vi "To String (Numeric).vi"(7 "enable LabVIEW extensions? (T)":bool=TRUE, 8 "error in (no error)":errorcluster, 11 "JSON Value in":refnum<class "JSON Value.lvclass">) -> (0 "error out":errorcluster, 3 "String":string)   [LabVIEW 2017, in "JSON Value.lvclass"]
doc: "Flattens the given JSON data to a string."
uses:
  JSON Value.lvclass
  JSON Value.lvclass/JSON Value.ctl
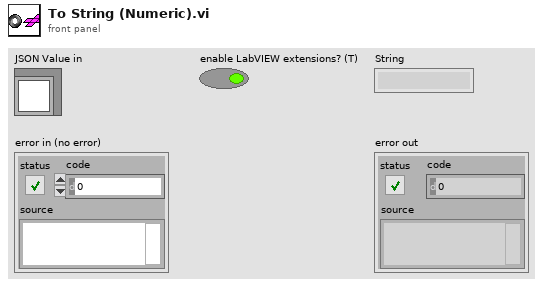
[diagram p1: front panel]
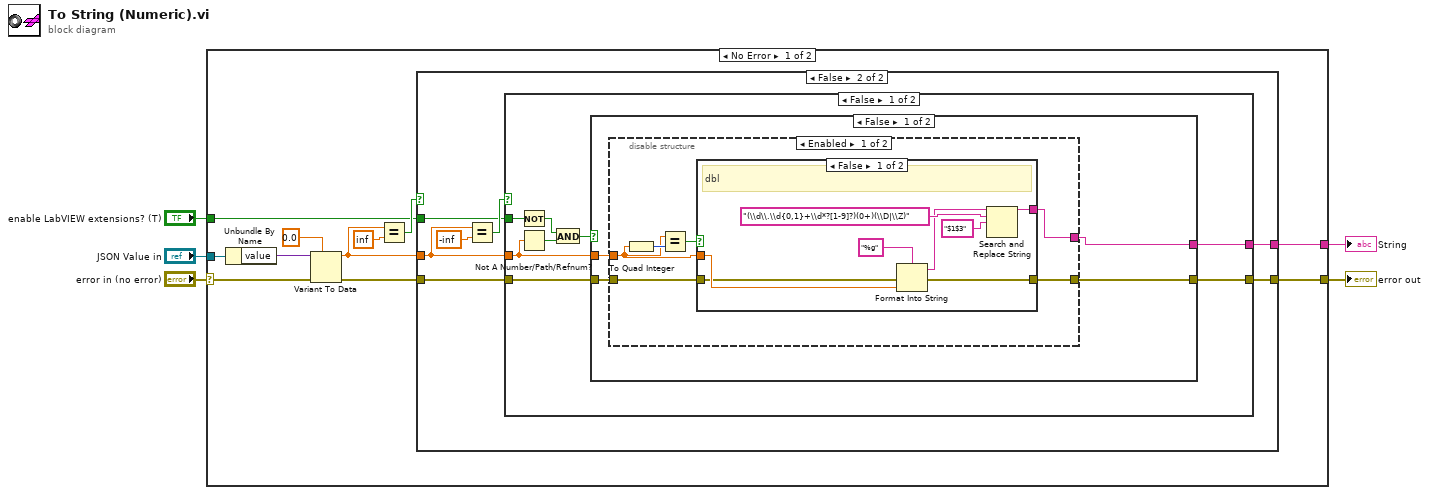
[diagram p0: block diagram]
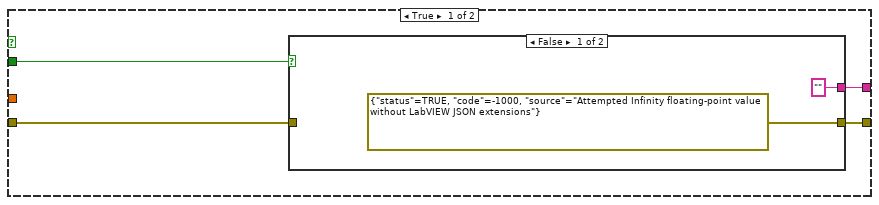
[diagram p2: hidden frame]
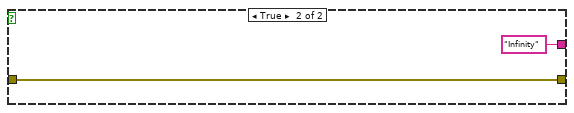
[diagram p3: hidden frame]
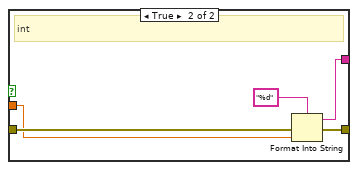
[diagram p4: hidden frame]
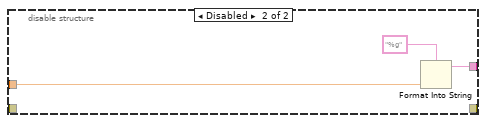
[diagram p5: hidden frame]
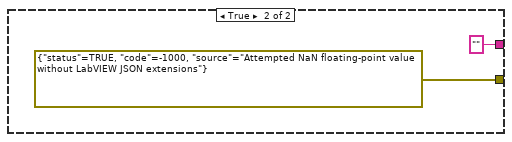
[diagram p6: hidden frame]
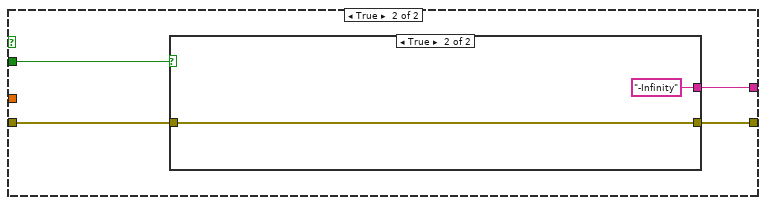
[diagram p7: hidden frame]
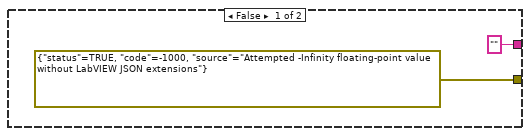
[diagram p8: hidden frame]
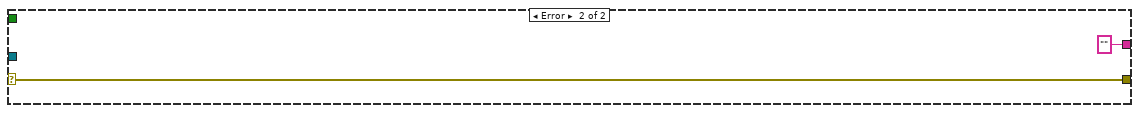
[diagram p9: hidden frame]
diagram:
  n1 = case shown="No Error" "error in (no error)" {
    selector: "error in (no error)" -> [w15 w77]
    tunnel: "JSON Value in" -> [w16 _]
    tunnel: [w14 ""] -> w3
    tunnel: [w13 w77] -> w2
    tunnel: "enable LabVIEW extensions? (T)" -> [w10 _]
    frame No Error {
      n2 = Unbundle By Name(w16) -> ("value"=w8:variant)
      n3 = Variant To Data(error in=w15, type=0.0 ("y"), Variant=w8) -> (data=w7:dbl, error out=w9:errorcluster)
      n4 = Equal?(x=w7, y=inf) -> (x = y?=w11:bool)
      n5 = case shown="False" w11 {
        tunnel: w9 -> [w18 w31]
        tunnel: [w20 w30] -> w14
        tunnel: [w17 w29] -> w13
        tunnel: w7 -> [_ w27]
        tunnel: w10 -> [w19 w25]
        frame True {
          n6 = case shown="False" w19 {
            tunnel: ["" "Infinity"] -> w20
            tunnel: w18 -> [_ w23]
            tunnel: [errorcluster {"status"=TRUE, "code"=-1000, "source"="Attempted Infinity floating-point value without LabVIEW JSON extensions"} ("error IO") w23] -> w17
            frame False {
            }
            frame True {
            }
          }
        }
        frame False {
          n7 = Equal?(x=w27, y=-inf) -> (x = y?=w26:bool)
          n8 = case shown="False" w26 {
            tunnel: w31 -> [w39 w69]
            tunnel: [w38 w70] -> w30
            tunnel: [w37 w71] -> w29
            tunnel: w27 -> [w33 _]
            tunnel: w25 -> [w35 w68]
            frame False {
              n9 = Not(x=w35) -> (.not. x?=w34:bool)
              n10 = Not A Number/Path/Refnum?(number/path/refnum=w33) -> (NaN/Path/Refnum?=w32:bool)
              n11 = And(x=w34, y=w32) -> (x .and. y?=w36:bool)
              n12 = case shown="False" w36 {
                tunnel: w39 -> [w43 _]
                tunnel: [w42 ""] -> w38
                tunnel: [w41 errorcluster {"status"=TRUE, "code"=-1000, "source"="Attempted NaN floating-point value without LabVIEW JSON extensions"} ("error IO")] -> w37
                tunnel: w33 -> [w40 _]
                frame False {
                  n13 = disable-structure shown="Enabled" {
                    disable-tunnel: w43 -> [w48 _]
                    disable-tunnel: [w47 w64] -> w42
                    disable-tunnel: [w46 _] -> w41
                    disable-tunnel: w40 -> [w44 w65]
                    frame Enabled {
                      n14 = To Quad Integer(1:w44) -> (0:w45:i64)
                      n15 = Equal?(x=w44, y=w45) -> (x = y?=w49:bool)
                      n16 = case shown="False" w49 {
                        tunnel: w48 -> [w55 w60]
                        tunnel: w44 -> [w57 w58]
                        tunnel: [w50 w61] -> w47
                        tunnel: [w54 w59] -> w46
                        frame False {
                          # "dbl"
                          n17 = Format Into String(format string="%g", error in=w55, w57) -> (resulting string=w51:string, error out=w54:errorcluster)  [unwired: 1 in]
                          n18 = Search and Replace String(input string=w51, search string="(\\d\\.\\d{0,1}+\\d*?[1-9]?)(0+)(\\D|\\Z)", replace string="$1$3" ("replace string (\"\")")) -> (result string=w50:string)  [unwired: 5 in, 3 out]
                        }
                        frame True {
                          # "int"
                          n19 = Format Into String(format string="%d", error in=w60, w58) -> (resulting string=w61:string, error out=w59:errorcluster)  [unwired: 1 in]
                        }
                      }
                    }
                    frame Disabled {
                      n20 = Format Into String(format string="%g", w65) -> (resulting string=w64:string)  [unwired: 2 in, 1 out]
                    }
                  }
                }
                frame True {
                }
              }
            }
            frame True {
              n21 = case shown="True" w68 {
                tunnel: ["" "-Infinity"] -> w70
                tunnel: w69 -> [_ w74]
                tunnel: [errorcluster {"status"=TRUE, "code"=-1000, "source"="Attempted -Infinity floating-point value without LabVIEW JSON extensions"} ("error IO") w74] -> w71
                frame False {
                }
                frame True {
                }
              }
            }
          }
        }
      }
    }
    frame Error {
    }
  }
  "String" <- w3
  "error out" <- w2
